vi "Credit Update.vi"(8 "error in (no error)":errorcluster, 10 "Credit":dbl, 11 "UI Actor in":refnum<class "UI Actor.lvclass">) -> (0 "error out":errorcluster, 3 "UI Actor out":refnum<class "UI Actor.lvclass">)   [LabVIEW 2020, in "UI Actor.lvlib" / "UI Actor.lvclass"]
uses:
  UI Actor.lvclass
  UI Actor.lvclass/UI Actor.ctl
  ESP Actor Messages/Update MSG Msg/Update MSG Msg.lvclass/Update MSG Msg.ctl
  <vilib>/ActorFramework/Message Enqueuer/Message Enqueuer.lvclass/Message Enqueuer.ctl
  <vilib>/ActorFramework/Message Enqueuer/Enqueue.vi
  ESP Actor Messages/Update MSG Msg/Update MSG Msg.lvclass
  C:/Program Files (x86)/National Instruments/LabVIEW 2020/vi.lib/ActorFramework/Message/Message.lvclass
  <vilib>/ActorFramework/Message Priority Queue/Priority Enqueue.vi
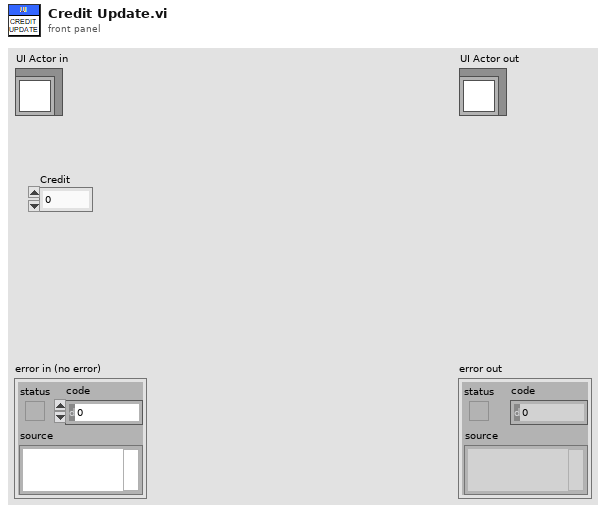
[diagram p1: front panel]
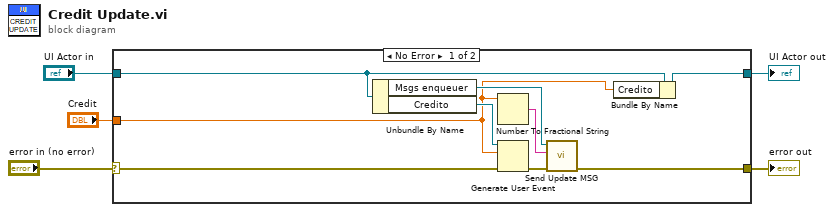
[diagram p0: block diagram]
diagram:
  n1 = case shown="No Error" "error in (no error)" {
    selector: "error in (no error)" -> [w14 w16]
    tunnel: [w8 w16] -> w4
    tunnel: [w7 w15] -> w2
    tunnel: "UI Actor in" -> [w13 w15]
    tunnel: "Credit" -> [w6 _]
    frame No Error {
      n2 = Unbundle By Name(w13) -> ("Msgs enqueuer"=w11:refnum<class "Message Enqueuer.lvclass">, "Credito"=w12:refnum<user-event>)
      n3 = Number To Fractional String(number=w6) -> (F-format string=w10:string)  [unwired: 3 in]
      n4 = Generate User Event(user event=w12, event data cluster=w6, error in=w14) -> (error out=w9:errorcluster)  [unwired: 1 in, 1 out]
      n5 = call "Send Update MSG.vi"("error in (no error)"=w9, "Update MSG"=w10, "Message Enqueuer"=w11) -> ("error out"=w8:errorcluster)  [unwired: 7 in, 1 out]
      n6 = Bundle By Name(cluster=w13, "Credito"=w6) -> (w7:refnum<class "UI Actor.lvclass">)
    }
    frame Error {
    }
  }
  "error out" <- w4
  "UI Actor out" <- w2
